vi "inertial simulation.vi"(3 "speeds":T3(array[cluster]) {"speed" step=0.05000000074505806 scale=-1.0..1.0; "turn" step=0.05000000074505806 scale=-1.0..1.0}, 4 "initial":T2, 5 "configuration":T5={"width (displayed)"=1.0, "actual width (m)"=1.0, "respect (none)"=enum."none", "iterations/s"=10.0, "maxiumum"={"speed"=1.5, "rotational acceleration"=0.2}, "coefficient of friction"={"forward"=0.04, "perpendicular"=0.08}, "robot start location"={"x"=0.0, "y"=0.0}}) -> (0 "locations":cluster{dbl, dbl}[](graph), 2 "output cluster":T1)   [LabVIEW 2009]
uses:
  arcade drive.llb/drive respect.ctl
panel:
  out "appended array":cluster{dbl[], dbl[]}[](graph)
  # "SPEED DOESN'T DESCELERATE PROPERLY\n(doesn't level out) WHEN \"turn\" is greater"
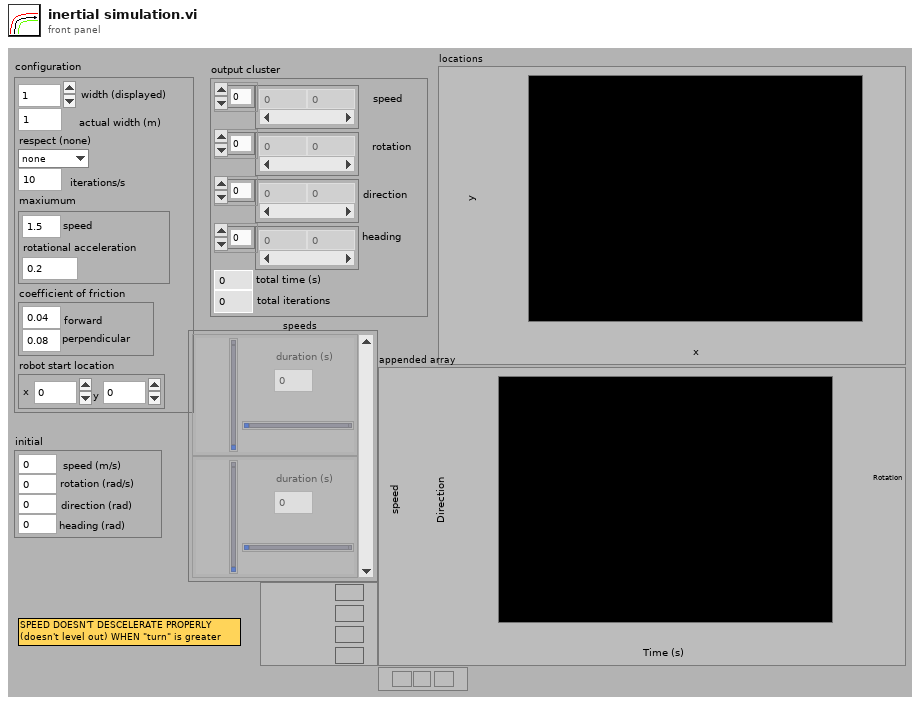
[diagram p1: front panel]
types:
  T1 = cluster{"speed":dbl[], "rotation":dbl[], "direction":dbl[], "heading":dbl[], "total time (s)":dbl, "total iterations":i32}
  T2 = cluster{"speed (m/s)":dbl, "rotation (rad/s)":dbl, "direction (rad)":dbl, "heading (rad)":dbl}
  T3 = cluster{"speed":dbl, "turn":dbl, "duration (s)":dbl}[]
  T4 = typedef "drive respect.ctl" = enum16{"none", "average", "turn", "speed"}
  T5 = cluster{"width (displayed)":dbl, "actual width (m)":dbl, "respect (none)":T4, "iterations/s":dbl, "maxiumum":cluster{"speed":dbl, "rotational acceleration":dbl}, "coefficient of friction":cluster{"forward":dbl, "perpendicular":dbl}, "robot start location":cluster{"x":dbl, "y":dbl}}
  T6 = cluster{"coefficient of friction":cluster{"forward":dbl, "perpendicular":dbl}, dbl}
  T7 = cluster{dbl[], dbl[], dbl[], dbl[], "duration (s)":dbl, i32}
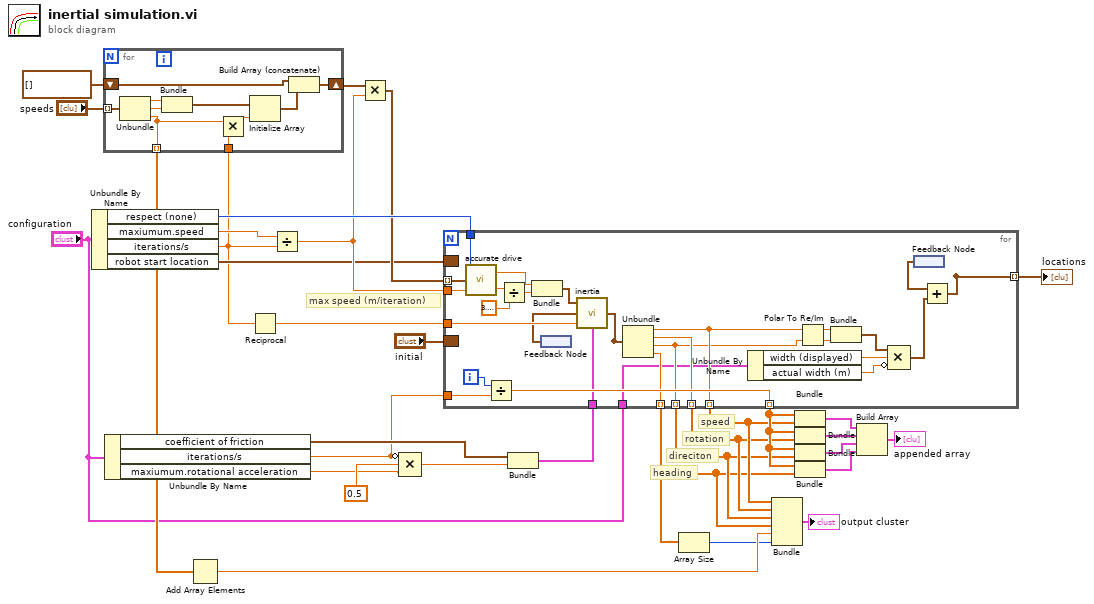
[diagram p0: block diagram]
diagram:
  # "heading"
  # "direciton"
  # "rotation"
  # "speed"
  # "max speed (m/iteration)"
  n1 = Unbundle By Name("configuration") -> ("respect (none)"=w31:T4, "maxiumum.speed"=w32:dbl, "iterations/s"=w25:dbl, "robot start location"=w26:cluster{"x":dbl, "y":dbl})
  n2 = for {
    tunnel: "speeds" -> [w43] mode=indexing
    tunnel: w25 -> [w40]
    shift-right: [w36] -> w6
    shift-left: cluster{"speed":dbl, "turn":dbl}[] [] -> [w35]
    tunnel: [w34] -> w12 mode=indexing
    n3 = Unbundle(w43) -> ("speed"=w42:dbl, "turn"=w41:dbl, "duration (s)"=w34:dbl)
    n4 = Bundle("speed"=w42, "turn"=w41) -> (w38:cluster{"speed":dbl, "turn":dbl})  [unwired: 1 in]
    n5 = Multiply(x=w34, y=w40) -> (x*y=w39:dbl)
    n6 = Initialize Array(w38, w39) -> (w37:cluster{"speed":dbl, "turn":dbl}[])
    n7 = Build Array (concatenate)(w35, w37) -> (w36:cluster{"speed":dbl, "turn":dbl}[])
  }
  n8 = Unbundle By Name("configuration") -> ("coefficient of friction"=w4:cluster{"forward":dbl, "perpendicular":dbl}, "iterations/s"=w3:dbl, "maxiumum.rotational acceleration"=w13:dbl)
  n9 = Add Array Elements(numeric array=w12) -> (sum=w8:dbl)
  n10 = Reciprocal(x=w25) -> (1/x=w24:dbl)
  n11 = Divide(x=w32, y=w25) -> (x/y=w27:dbl)
  n12 = Multiply(x=w6, y=w27) -> (x*y=w28:cluster{"speed":dbl, "turn":dbl}[])
  n13 = Compound Arithmetic op=MULTIPLY(invert w3, 0.5, w13) -> (w21:dbl)
  n14 = Bundle("coefficient of friction"=w4, w21) -> (w22:T6)  [unwired: 1 in]
  n15 = for {
    tunnel: [w45] -> w33 mode=indexing
    tunnel: w27 -> [w68]
    tunnel: w31 -> [w63]
    tunnel: w28 -> [w67] mode=indexing
    tunnel: w3 -> [w65]
    tunnel: [w51] -> w11 mode=indexing
    tunnel: [w64] -> w20 mode=indexing
    tunnel: [w52] -> w10 mode=indexing
    tunnel: w24 -> [w56]
    border: "initial" -> [_]
    tunnel: [w53] -> w1 mode=indexing
    border: w26 -> [_]
    tunnel: [w50] -> w9 mode=indexing
    tunnel: w22 -> [w49]
    tunnel: "configuration" -> [w48]
    i -> [w66]
    n16 = call "accurate drive.vi"("range"=w68, "speeds"=w67, "respect turn? (respect speed)"=w63) -> ("speed"=w60:dbl, "turn"=w58:dbl)  [unwired: 1 out]
    n17 = Divide(x=w66, y=w65) -> (x/y=w64:dbl)
    n18 = Divide(x=w60, y=3.141592653589793) -> (x/y=w59:dbl)
    n19 = Bundle("turn"=w58, w59) -> (w57:cluster{"turn":dbl, dbl})  [unwired: 1 in]
    n20 = feedback #1() -> (w54:T2)
    n21 = call "inertia.vi"("constants"=w49, "time elapsed (s)"=w56, "residual"=w54, "applied"=w57) -> ("estimated"=w55:T2)
    n22 = Unbundle(w55) -> ("speed (m/s)"=w51:dbl, "rotation (rad/s)"=w52:dbl, "direction (rad)"=w50:dbl, "heading (rad)"=w53:dbl)
    n23 = Unbundle By Name(w48) -> ("width (displayed)"=w47:dbl, "actual width (m)"=w46:dbl)
    n24 = Polar To Re/Im(2:w50, 3:w51) -> (0:w71:dbl, 1:w70:dbl)
    n25 = Bundle(w70, w71) -> (w62:cluster{dbl, dbl})  [unwired: 1 in]
    n26 = Compound Arithmetic op=MULTIPLY(w62, w47, invert w46) -> (w61:cluster{dbl, dbl})
    n27 = feedback #2() -> (w44:cluster{"x":dbl, "y":dbl})
    n28 = Add(x=w44, y=w61) -> (x+y=w45:cluster{dbl, dbl})
  }
  "locations" <- w33
  n29 = Array Size(array=w1) -> (size(s)=w5:i32)
  n30 = Bundle(w11, w10, w9, w1, "duration (s)"=w8, w5) -> (→"output cluster":T7)  [unwired: 1 in]
  n31 = Bundle(w20, w11) -> (w16:cluster{dbl[], dbl[]})  [unwired: 1 in]
  n32 = Bundle(w20, w10) -> (w17:cluster{dbl[], dbl[]})  [unwired: 1 in]
  n33 = Bundle(w20, w9) -> (w18:cluster{dbl[], dbl[]})  [unwired: 1 in]
  n34 = Bundle(w20, w1) -> (w19:cluster{dbl[], dbl[]})  [unwired: 1 in]
  n35 = Build Array(w16, w17, w18, w19) -> (→"appended array":cluster{dbl[], dbl[]}[])
